vi "Invoke Measure Logic.vi"(8 "error in":errorcluster, 10 "gRPCid in":T1, 11 "gRPC Server in":refnum<class "MeasurementService.lvclass">) -> (0 "error out":errorcluster)   [LabVIEW 2020, in "MeasurementLink Measurement Server.lvlib" / "MeasurementService.lvclass"]
uses:
  MeasurementService.lvclass
  <vilib>/gRPC/LabVIEW gRPC Library/Shared/grpcId.ctl
  <vilib>/gRPC/LabVIEW gRPC Library/Server API/typeDefs/gRPC Status Code.ctl
  MeasurementContext/MeasurementContext.lvclass
  <vilib>/gRPC/LabVIEW gRPC Library/grpc-lvsupport-release.lvlib
  MeasurementLink Measurement Server Internal/RPC Service/MeasurementService/MeasurementService.lvclass
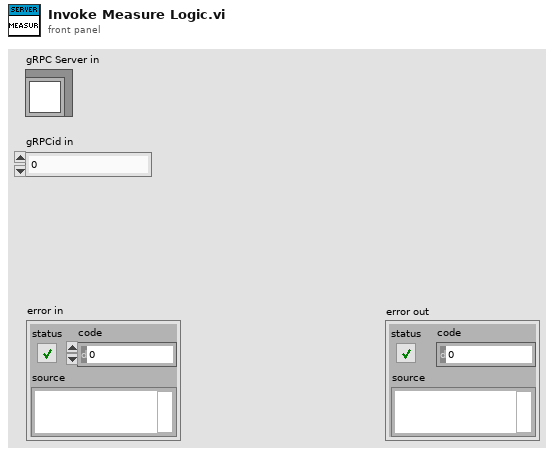
[diagram p1: front panel]
types:
  T1 = typedef "grpc-lvsupport-release.lvlib/grpcId.ctl" = u64
  T2 = typedef "MeasurementLink Measurement Server Internal.lvlib/ni_measurementlink_measurement_v1_MeasureRequest.ctl" = cluster{"configuration_parameters":T3, "pin_map_context":T4}
  T3 = typedef "MeasurementLink Measurement Server Internal.lvlib/google_protobuf_Any.ctl" = cluster{"type_url":string, "value":u8[]}
  T4 = typedef "MeasurementLink Measurement Server Internal.lvlib/ni_measurementlink_PinMapContext.ctl" = cluster{"pin_map_id":string, "sites":i32[]}
  T5 = typedef "grpc-lvsupport-release.lvlib/gRPC Status Code.ctl" = enum16{"OK", "CANCELLED", "UNKNOWN", "INVALID_ARGUMENT", "DEADLINE_EXCEEDED", "NOT_FOUND", "ALREADY_EXISTS", "PERMISSION_DENIED", "RESOURCE_EXHAUSTED", "FAILED_PRECONDITION", "ABORTED", "OUT_OF_RANGE", "UNIMPLEMENTED", "INTERNAL", "UNAVAILABLE", "DATA_LOSS", "UNAUTHENTICATED"}
  T6 = typedef "grpc-lvsupport-release.lvlib/Any.ctl" = cluster{"Type Url":string, "Bytes":u8[]}
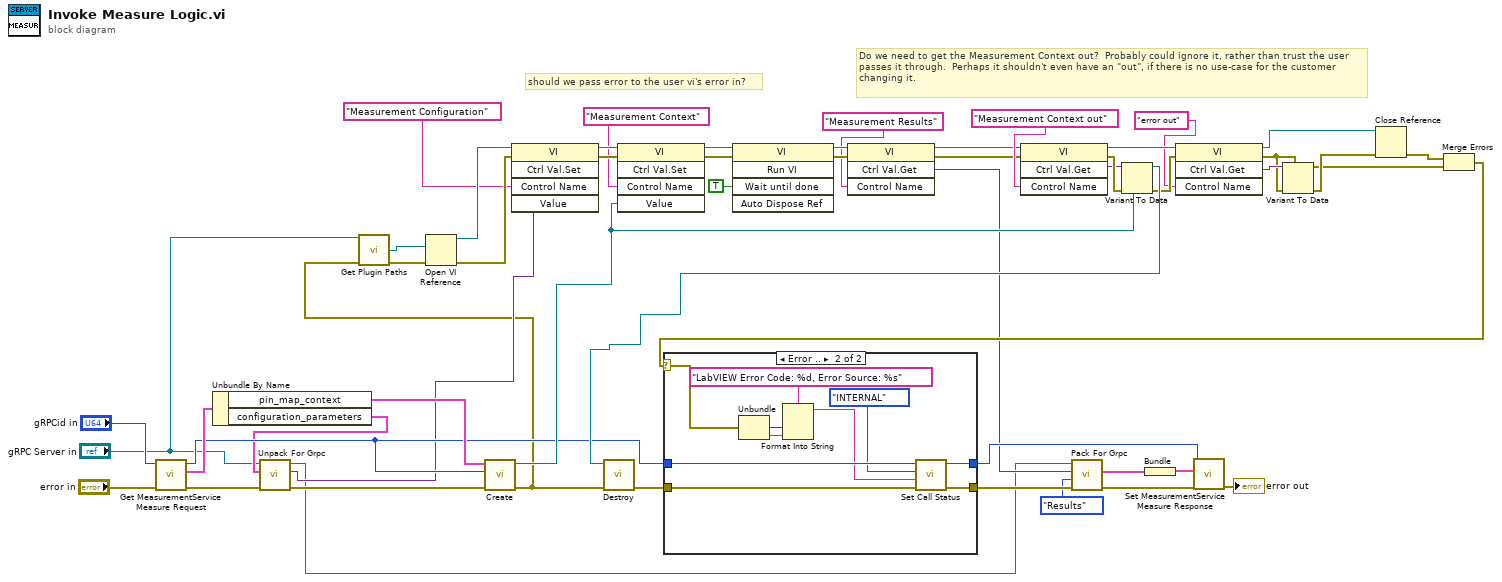
[diagram p0: block diagram]
diagram:
  # "should we pass error to the user vi's error in?"
  # "Do we need to get the Measurement Context out?  Probably could ignore it, rather than trust the user passes it through.  Perhaps it shouldn't even have an \"out\", if there is no use-case for the customer changing it."
  n1 = call "Get MeasurementService Measure Request.vi"("error in (no error)"="error in", "gRPCid in"="gRPCid in") -> ("error out"=w16:errorcluster, "Message Data"=w50:T2, "gRPCid out"=w17:T1)  [unwired: 7 in]
  n2 = Unbundle By Name(w50) -> ("pin_map_context"=w49:T4, "configuration_parameters"=w15:T3)
  n3 = call-dynamic "Unpack For Grpc.vi"("error in (no error)"=w16, "Any"=w15, "gRPC Server in"="gRPC Server in") -> ("error out"=w13:errorcluster, "Data Value"=w14:variant, "gRPC Server out"=w5:refnum<class "MeasurementService.lvclass">)  [unwired: 6 in]
  n4 = call "Create.vi"("error in (no error)"=w13, "gRPC server call"=w17, "pin map context"=w49) -> ("error out"=w3:errorcluster, "MeasurementContext out"=w30:refnum<class "MeasurementContext.lvclass">)  [unwired: 7 in]
  n5 = call-dynamic "Get Plugin Paths.vi"("MeasurementService in"="gRPC Server in", "error in (no error)"=w3) -> ("Measurement Logic VI Path"=w2:path, "error out"=w4:errorcluster)  [unwired: 7 in, 5 out]
  n6 = Open VI Reference(vi path=w2, error in (no error)=w4) -> (vi reference=w45:refnum<vi>, error out=w44:errorcluster)  [unwired: 4 in]
  n7 = invoke class="VI" method="Ctrl Val.Set"(reference=w45, error in=w44, "Control Name"="Measurement Configuration", "Value"=w14) -> (reference out=w42:refnum<vi>, error out=w41:errorcluster)  [unwired: 1 in, 3 out]
  n8 = invoke class="VI" method="Ctrl Val.Set"(reference=w42, error in=w41, "Control Name"="Measurement Context", "Value"=w30) -> (reference out=w38:refnum<vi>, error out=w39:errorcluster)  [unwired: 1 in, 3 out]
  n9 = invoke class="VI" method="Run VI"(reference=w38, error in=w39, "Wait until done"=TRUE ("Wait Until Done")) -> (reference out=w36:refnum<vi>, error out=w35:errorcluster)  [unwired: 2 in, 3 out]
  n10 = invoke class="VI" method="Ctrl Val.Get"(reference=w36, error in=w35, "Control Name"="Measurement Results") -> (reference out=w28:refnum<vi>, error out=w19:errorcluster, "Get Control Value Variant"=w9:variant)  [unwired: 1 in, 1 out]
  n11 = invoke class="VI" method="Ctrl Val.Get"(reference=w28, error in=w19, "Control Name"="Measurement Context out") -> (reference out=w27:refnum<vi>, error out=w32:errorcluster, "Get Control Value Variant"=w31:variant)  [unwired: 1 in, 1 out]
  n12 = Variant To Data(error in=w32, type=w30, Variant=w31) -> (data=w29:refnum<class "MeasurementContext.lvclass">, error out=w26:errorcluster)
  n13 = call-dynamic "Destroy.vi"("error in (no error)"=w3, "MeasurementContext in"=w29) -> ("error out"=w48:errorcluster)  [unwired: 9 in]
  n14 = invoke class="VI" method="Ctrl Val.Get"(reference=w27, error in=w26, "Control Name"="error out") -> (reference out=w23:refnum<vi>, error out=w22:errorcluster, "Get Control Value Variant"=w24:variant)  [unwired: 1 in, 1 out]
  n15 = Variant To Data(error in=w22, type=w22, Variant=w24) -> (data=w20:errorcluster, error out=w21:errorcluster)
  n16 = Close Reference(reference=w23, error in (no error)=w21) -> (error out=w47:errorcluster)
  n17 = Merge Errors(w47, w20) -> (w46:errorcluster)
  n18 = case shown="Error .." w46 {
    selector: w46 -> [_ w64]
    tunnel: w17 -> [w54 w63]
    tunnel: [w54 w62] -> w18
    tunnel: w48 -> [w53 w60]
    tunnel: [w53 w61] -> w12
    frame No Error {
    }
    frame Error {
      n19 = Unbundle(w64) -> ("code"=w58:i32, "source"=w57:string)  [unwired: 1 out]
      n20 = Format Into String(format string="LabVIEW Error Code: %d, Error Source: %s", w58, w57) -> (resulting string=w55:string)  [unwired: 2 in, 1 out]
      n21 = call <vilib>:"Set Call Status.vi"("error in"=w60, "Details"=w55, "Status Code"=gRPC_Status_Code."INTERNAL", "gRPCid in"=w63) -> ("error out"=w61:errorcluster, "gRPCid out"=w62:T1)  [unwired: 6 in]
    }
  }
  n22 = call-dynamic "Pack For Grpc.vi"("error in (no error)"=w12, "Configuration / Resuls (Config)"=enum16{"Configuration", "Results"}."Results", "Data Value"=w9, "gRPC Server in"=w5) -> ("error out"=w8:errorcluster, "Any"=w10:T6)  [unwired: 5 in, 1 out]
  n23 = Bundle("Any"=w10) -> (w52:cluster{"Any":T6})  [unwired: 1 in]
  n24 = call "Set MeasurementService Measure Response.vi"("error in (no error)"=w8, "Message Data"=w52, "gRPCid in"=w18) -> ("error out"=→"error out":errorcluster)  [unwired: 8 in]
